vi "GetPrivateQueueAction.vi"(8 "error in (no error)":errorcluster, 11 "Generator":refnum<class "Generator.lvclass">) -> (0 "error out":errorcluster, 3 "Generator out":refnum<class "Generator.lvclass">)   [LabVIEW 2019, in "Generator.lvclass"]
uses:
  Generator.lvclass
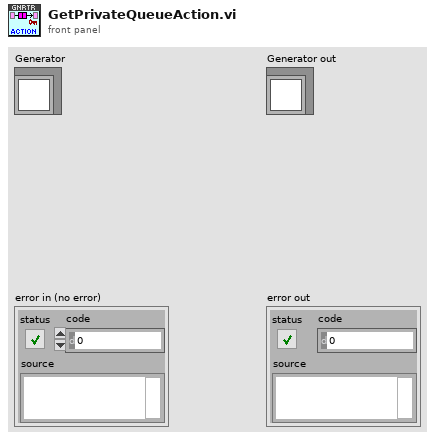
[diagram p1: front panel]
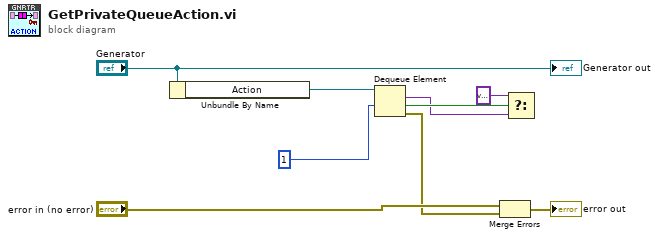
[diagram p0: block diagram]
diagram:
  n1 = Unbundle By Name("Generator") -> ("Action"=w9:refnum<queue>)
  n2 = Dequeue Element(queue=w9, timeout in ms (-1)=1) -> (element=w4:variant, timed out?=w8:bool, error out=w6:errorcluster)  [unwired: 1 in, 1 out]
  n3 = Merge Errors("error in (no error)", w6) -> (→"error out":errorcluster)
  n4 = Select(t=variant, s=w8, f=w4) -> ()  [unwired: 1 out]
  "Generator out" <- "Generator"
